vi "Get Static (Func Global).vi"(8 "error in (no error)":errorcluster, 11 "Numeric in":refnum<class "Numeric Test Object.lvclass">) -> (0 "error out":errorcluster, 2 "Int":i32, 3 "Numeric out":refnum<class "Numeric Test Object.lvclass">)   [LabVIEW 2009, in "Numeric Test Object.lvclass"]
doc: "Gets the static data held in the functional global."
uses:
  Numeric Test Object.lvclass
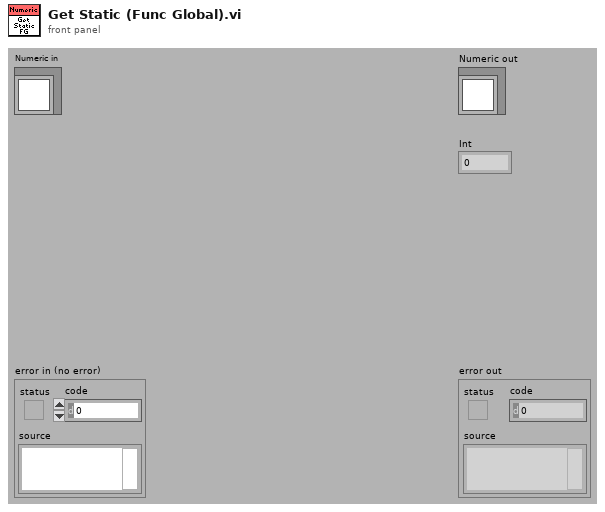
[diagram p1: front panel]
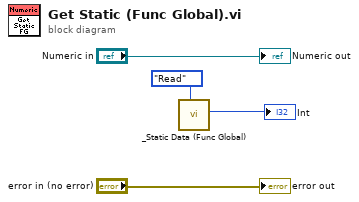
[diagram p0: block diagram]
diagram:
  n1 = call "_Static Data (Func Global).vi"("Function (Read)"=enum16{"Read", "Write"}."Read") -> ("Numeric out"=→"Int":i32)  [unwired: 8 in, 2 out]
  "error out" <- "error in (no error)"
  "Numeric out" <- "Numeric in"
